vi "AIDI-Read (AI).vi"(0 "Tasks In":T1[](array[typedef]), 7 "number of samples per channel":i32=-1, 11 "error in (no error)":errorcluster) -> (4 "Tasks Out":T1[](array[typedef]), 8 "AO Waveforms":dbl[][](array[numeric]), 15 "error out":errorcluster)   [LabVIEW 2020]
uses:
  Typedefs/AIDI-Task Specification.ctl
  <vilib>/DAQmx/read.llb/DAQmx Read (Analog 2D DBL NChan NSamp).vi
  <vilib>/DAQmx/read.llb/DAQmx Read (Analog 1D DBL 1Chan NSamp).vi
  <vilib>/DAQmx/miscellaneous.llb/DAQmx Fill In Error Info.vi
panel:
  in  "timeout":dbl=10.0 format="%#_13g"
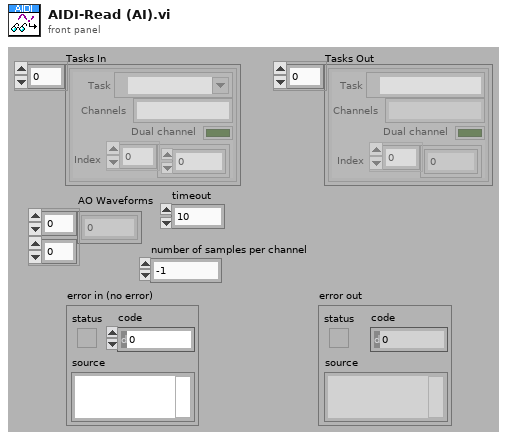
[diagram p1: front panel]
types:
  T1 = typedef "AIDI-Task Specification.ctl" = cluster{"Task":refnum<k21>, "Channels":string, "Dual channel":bool, "Index":i32[]}
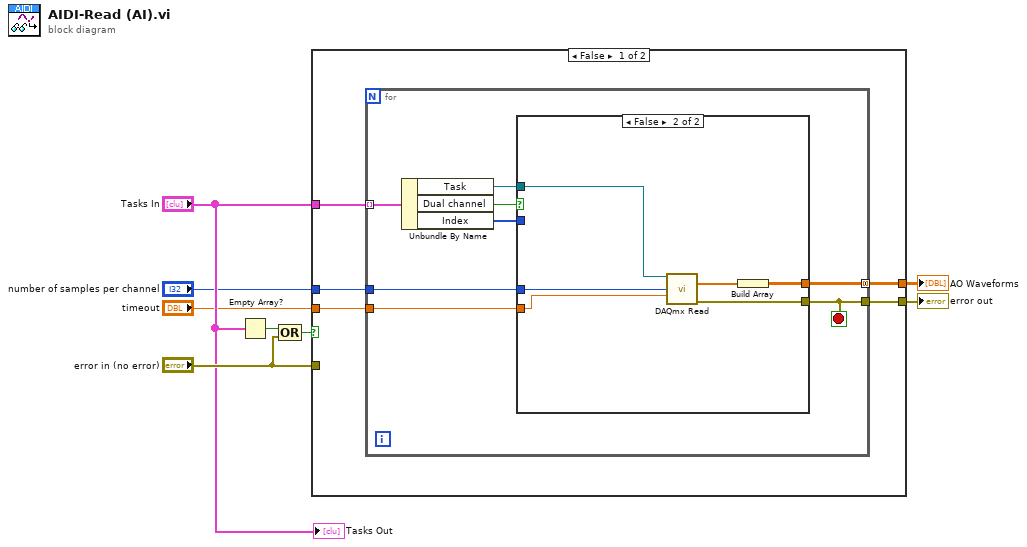
[diagram p0: block diagram]
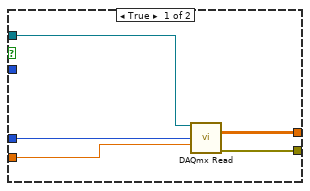
[diagram p2: hidden frame]
diagram:
  n1 = Empty Array?(array="Tasks In") -> (empty?=w5:bool)
  n2 = Compound Arithmetic op=OR(w5, "error in (no error)") -> (w7:bool)
  n3 = case shown="False" w7 {
    tunnel: [w13 w33] -> w8
    tunnel: "error in (no error)" -> [_ w33]
    tunnel: "Tasks In" -> [w12 _]
    tunnel: [w11 _] -> w3
    tunnel: "number of samples per channel" -> [w10 _]
    tunnel: "timeout" -> [w9 _]
    frame False {
      n4 = for {
        tunnel: w12 -> [w20] mode=indexing
        tunnel: [w14] -> w13
        tunnel: [w17] -> w11 mode=concatenating
        tunnel: w10 -> [w16]
        tunnel: w9 -> [w15]
        stop <- w14 stop-if-true
        n5 = Unbundle By Name(w20) -> ("Task"=w19:refnum<k21>, "Dual channel"=w21:bool, "Index"=w18:i32[])
        n6 = case shown="False" w21 {
          tunnel: w19 -> [w25 w31]
          tunnel: [w26 w32] -> w14
          tunnel: w18 -> [_ _]
          tunnel: [w24 w29] -> w17
          tunnel: w16 -> [w23 w28]
          tunnel: w15 -> [w22 w27]
          frame True {
            n7 = call-poly <vilib>:"DAQmx Read.vi"("task/channels in"=w25, "number of samples per channel"=w23, "timeout"=w22) -> ("data"=w24:dbl[][], "error out"=w26:errorcluster)  [unwired: 10 in, 1 out]
          }
          frame False {
            n8 = call-poly <vilib>:"DAQmx Read.vi"("task/channels in"=w31, "number of samples per channel"=w28, "timeout"=w27) -> ("data"=w30:dbl[], "error out"=w32:errorcluster)  [unwired: 10 in, 1 out]
            n9 = Build Array(w30) -> (w29:dbl[][])
          }
        }
      }
    }
    frame True {
    }
  }
  "error out" <- w8
  "AO Waveforms" <- w3
  "Tasks Out" <- "Tasks In"
